vi "Custom - Zero.vi"(8 "error in (no error)":errorcluster, 11 "Address":string) -> (0 "error out":errorcluster, 2 "Calibration Success":bool)   [LabVIEW 2025, in "Interface Functions.lvlib"]
uses:
  Interface Functions.lvlib
  <instrlib>/Agilent U2000 Series/Agilent U2000 Series.lvlib
panel:
  # "Custom - Zero Sensor"
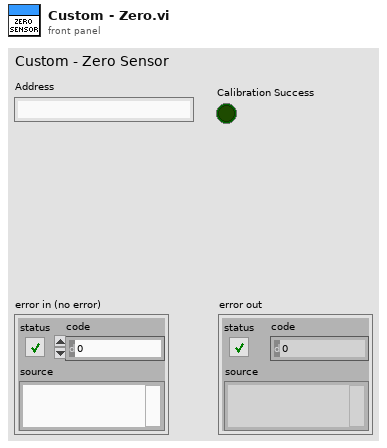
[diagram p1: front panel]
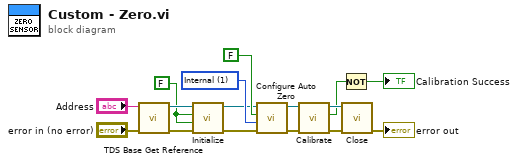
[diagram p0: block diagram]
diagram:
  w3 = FALSE ("ID Query (True)")
  w13 = 1 items=["External", "Internal"] ("Zero Type (0: External)")
  n1 = call "TDS Base Get Reference.vi"("error in (no error)"="error in (no error)", "Address"="Address") -> ("error out"=w7:errorcluster, "Reference"=w4:refnum<visa-resource-name>)  [unwired: 8 in]
  n2 = call <instrlib>:"Initialize.vi"("error in (no error)"=w7, "Reset (True)"=w3, "ID Query (True)"=w3, "VISA resource name"=w4) -> ("error out"=w6:errorcluster, "VISA resource name out"=w5:refnum<visa-resource-name>)  [unwired: 6 in]
  n3 = call <instrlib>:"Configure Auto Zero.vi"("error in (no error)"=w6, "Zero Type (0: External)"=w13, "Auto Zero (T: Enable)"=FALSE, "VISA resource name"=w5) -> ("error out"=w12:errorcluster, "VISA resource name out"=w11:refnum<visa-resource-name>)  [unwired: 6 in]
  n4 = call <instrlib>:"Calibrate.vi"("error in (no error)"=w12, "VISA resource name"=w11) -> ("error out"=w10:errorcluster, "Calibration Result"=w1:bool, "VISA resource name out"=w9:refnum<visa-resource-name>)  [unwired: 7 in]
  n5 = Not(x=w1) -> (.not. x?=→"Calibration Success":bool)
  n6 = call <instrlib>:"Close.vi"("error in (no error)"=w10, "VISA resource name"=w9) -> ("error out"=→"error out":errorcluster)  [unwired: 9 in]
